vi "Lectura Inventario.vi"(8 "error in":errorcluster) -> (0 "error out":errorcluster, 3 "Inventario":string[][](array[string]))   [LabVIEW 2024, in "ProductControl.lvlib"]
uses:
  ProductControl.lvlib
  <vilib>/Utility/config.llb/Read Key (String).vi
  <vilib>/Utility/config.llb/NI_LVConfig.lvlib
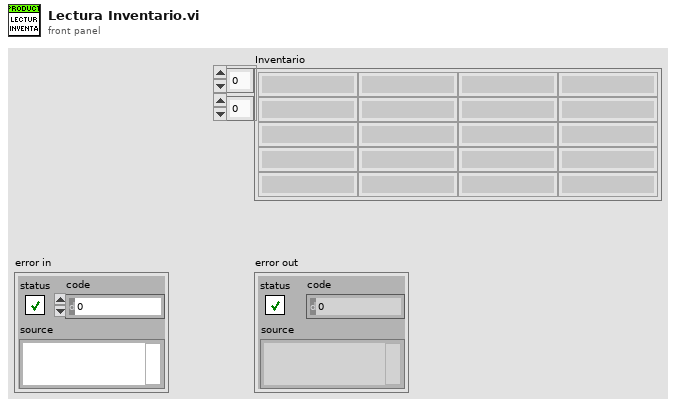
[diagram p1: front panel]
types:
  T1 = typedef "NI_LVConfig.lvlib/Config Data RefNum.ctl" = refnum<k1>
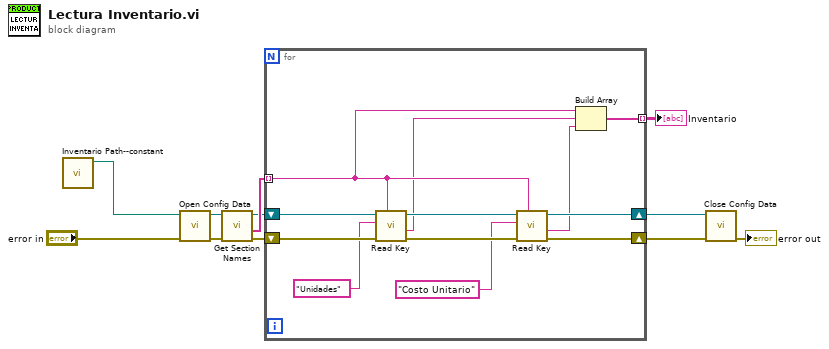
[diagram p0: block diagram]
diagram:
  n1 = call "Inventario Path--constant.vi"() -> ("Ruta Inventario"=w2:path)  [unwired: 11 in]
  n2 = call <vilib>:"Open Config Data.vi"("error in (no error)"="error in", "configuration file path"=w2) -> ("error out"=w11:errorcluster, "refnum"=w6:T1)  [unwired: 7 in, 1 out]
  n3 = call <vilib>:"Get Section Names.vi"("error in (no error)"=w11, "refnum"=w6) -> ("error out"=w10:errorcluster, "section names"=w5:string[], "refnum out"=w4:T1)  [unwired: 7 in]
  n4 = for {
    tunnel: w5 -> [w15] mode=indexing
    shift-right: [w17] -> w3
    shift-left: w4 -> [w19]
    shift-right: [w21] -> w9
    shift-left: w10 -> [w23]
    tunnel: [w12] -> w1 mode=indexing
    n5 = call-poly <vilib>:"Read Key.vi"("section"=w15, "error in (no error)"=w23, "key"="Unidades", "refnum"=w19) -> ("error out"=w22:errorcluster, "value"=w14:string, "refnum out"=w18:T1)  [unwired: 4 in, 1 out]
    n6 = call-poly <vilib>:"Read Key.vi"("section"=w15, "error in (no error)"=w22, "key"="Costo Unitario", "refnum"=w18) -> ("error out"=w21:errorcluster, "value"=w13:string, "refnum out"=w17:T1)  [unwired: 4 in, 1 out]
    n7 = Build Array(w15, w14, w13) -> (w12:string[])
  }
  "Inventario" <- w1
  n8 = call <vilib>:"Close Config Data.vi"("error in (no error)"=w9, "refnum"=w3) -> ("error out"=→"error out":errorcluster)  [unwired: 8 in, 1 out]
